vi "POSCAR Structure array to GULP.vi"() -> ()   [LabVIEW 2010]
panel:
  in  "Path":path
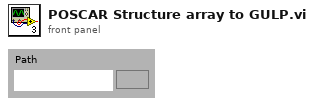
[diagram p1: front panel]
types:
  T1 = cluster{"Structure Name":string, "Lattice vector a":dbl[], "Lattice vector b":dbl[], "Lattice vector c":dbl[], "Atoms Array":cluster{"Atom Name":string, "Positions (Direct)":dbl[][], "Positions (Cartesian)":dbl[][]}[], "# of atoms":i32}
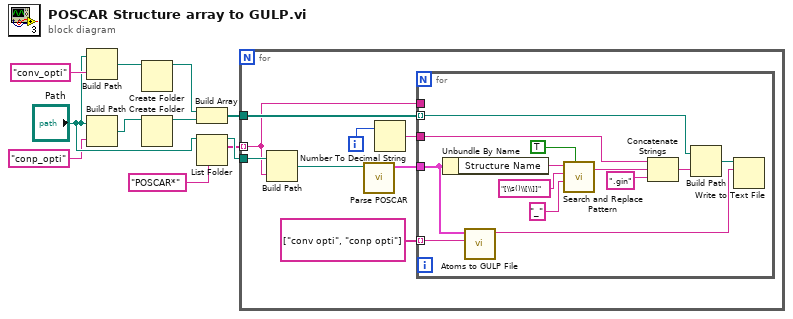
[diagram p0: block diagram]
diagram:
  n1 = Build Path(base path="Path", name or relative path="conv_opti") -> (appended path=w8:path)
  n2 = Build Path(base path="Path", name or relative path="conp_opti") -> (appended path=w6:path)
  n3 = Create Folder(path (use dialog)=w8) -> (created path=w3:path)  [unwired: 2 in, 2 out]
  n4 = Create Folder(path (use dialog)=w6) -> (created path=w2:path)  [unwired: 2 in, 2 out]
  n5 = Build Array(w3, w2) -> (w1:path[])
  n6 = List Folder(path="Path", pattern="POSCAR*") -> (path out=w11:path, filenames=w10:string[])  [unwired: 2 in, 2 out]
  n7 = for {
    tunnel: w11 -> [w19]
    tunnel: w10 -> [w14] mode=indexing
    tunnel: w1 -> [w15]
    i -> [w13]
    n8 = Build Path(base path=w19, name or relative path=w14) -> (appended path=w18:path)
    n9 = call "Parse POSCAR.vi"("POSCAR File"=w18) -> ("Structure"=w17:T1)  [unwired: 7 in, 3 out]
    n10 = Number To Decimal String(number=w13) -> (decimal integer string=w12:string)  [unwired: 1 in]
    n11 = for {
      tunnel: w17 -> [w26]
      tunnel: string[] ["conv opti", "conp opti"] -> [w32] mode=indexing
      tunnel: w15 -> [w30] mode=indexing
      tunnel: w14 -> [_]
      tunnel: w12 -> [w27]
      n12 = Unbundle By Name(w26) -> ("Structure Name"=w21:string)
      n13 = call "Atoms to GULP File.vi"("Relaxation Type"=w32, "Structure"=w26) -> ("GULP File"=w31:string)  [unwired: 9 in]
      n14 = call <vilib>:"Search and Replace Pattern.vi"("string"=w21, "regular expression (\"\")"="[\\s()\\[\\]]" ("regular expression (\"\")"), "replace string (\"\")"="_" ("replace string (\"\")"), "replace all? (F)"=TRUE) -> ("result string"=w20:string)  [unwired: 1 in, 1 out]
      n15 = Concatenate Strings(w27, w20, ".gin" ("string")) -> (w25:string)
      n16 = Build Path(base path=w30, name or relative path=w25) -> (appended path=w28:path)
      n17 = Write to Text File(file (use dialog)=w28, text=w31) -> ()  [unwired: 2 in, 3 out]
    }
  }
